vi "Pointer.Read (1D SGL).vi"(8 "error in (no error)":errorcluster, 10 "count":i32, 11 "pointer in":u64) -> (0 "error out":errorcluster, 2 "values":sgl[](array[numeric]), 3 "pointer out":u64)   [LabVIEW 2016, in "VeriStand Data.lvlib"]
doc: "Reads a number of values, specified by <B>count</B>, from the provided <B>pointer</B>."
uses:
  VeriStand Data.lvlib
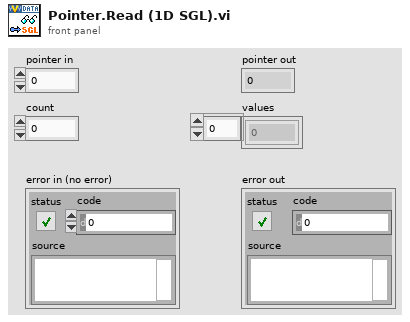
[diagram p1: front panel]
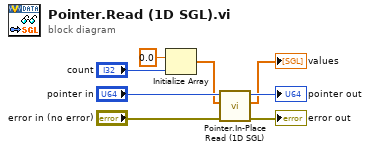
[diagram p0: block diagram]
diagram:
  n1 = Initialize Array(sgl 0.0 ("element"), "count") -> (w1:sgl[])
  n2 = call "Pointer.In-Place Read (1D SGL).vi"("error in (no error)"="error in (no error)", "allocated array in"=w1, "pointer in"="pointer in") -> ("error out"=→"error out":errorcluster, "array out"=→"values":sgl[], "pointer out"=→"pointer out":u64)  [unwired: 6 in]
